vi "Mercury_GCS_All_VIs.vi"   [LabVIEW 2011]
doc: "This VI contains all high level and low level VIs valid for Mercury_GCS. See diagram for a survey of all Mercury_GCS high level and low level VIs. Menu / Browse / Show VI Hierarchy will show the file paths of the VIs. Global Variables are shown as Control as well as Indicator."
uses:
  Low Level/General command.llb/Controller names.ctl
  Low Level/Communication.llb/Available DLL interfaces.ctl
  Low Level/Communication.llb/Available DLLs.ctl
  Low Level/Communication.llb/Available interfaces.ctl
  Low Level/Communication.llb/Termination character.ctl
  Low Level/Analog control.llb/Available Analog Commands.ctl
  Low Level/Communication.llb/Global1.vi
  Low Level/General command.llb/Global2 (Array).vi
  Low Level/Communication.llb/Global DaisyChain.vi
  Low Level/Analog control.llb/Global Analog.vi
  Low Level/Support.llb/Unbunde/bundle interface clusters for PI Terminal.vi
panel:
  # "PI Mercury_GCS \nLabVIEW driver set"
  # "This VI contains all high level and low level VIs valid for Mercury_GCS. See diagram for a\nsurvey of all Mercury_GCS high level and low level VIs. Menu / Browse / Show VI \nhierarchy will show the file paths of the VIs. Global Variables are shown as Control as \nwell as Indicator."
types:
  T1 = typedef "Available Analog Commands.ctl" = enum16{"INITIALIZE", "VOL?", "VOL ", "CLOSE", "MOV", "POS?", "VCO", "VCO?", "WAIT_WF", "TMN?", "TMX?", "VEL", "VEL?", "SAI?", "MVR", "ERR?", "#24", "STP", "*IDN?", "#5", "STE", "DRR?", "W_Wave", "HLP?", "W/R_Wave"}
  T2 = typedef "Termination character.ctl" = enum16{"LF", "CR", "LFCR", "CRLF"}
  T3 = typedef "Available interfaces.ctl" = u16
  T4 = typedef "Available DLLs.ctl" = u16
  T5 = typedef "Available DLL interfaces.ctl" = u16
  T6 = typedef "Controller names.ctl" = enum16{"None", "Analog", "C-702", "C-843", "C-843.PM", "C-844", "C-848", "C-865", "C-866", "C-867", "C-880", "E-516", "E-517", "E-709", "E-710", "E-712", "E-725", "E-753", "E-755", "E-761", "E-816", "E-861", "F-206", "M-840", "M-850", "M-8X0", "Mercury", "Mercury_GCS"}
  T7 = cluster{"Conversion factor":dbl[], "Velocity":dbl[], "Velocity control mode":bool, "AO.Resolution":dbl, "Lower voltage limit (V)":dbl, "Upper voltage limit (V)":dbl, "AO_WF_T (s)":dbl, "AI Sample Rate":dbl, "AI Samples/Channel":i32, "Hyperbit":bool, "Offset (V)":dbl[], "Hyperbit StayOnPos":bool, "Gain (V)":dbl[], "Bit rate (Hz)":dbl, "PWM rate (Hz)":dbl, "HyperBit Password":string, "AO.MaxRate":dbl, "Conversion offset":dbl[]}[]
  T8 = cluster{"No. of devices":i32, "Port ID":i32, "Devices":string[], "Description":string}[]
  T9 = cluster{"Conn. axes":string[], "Controller name":T6}[]
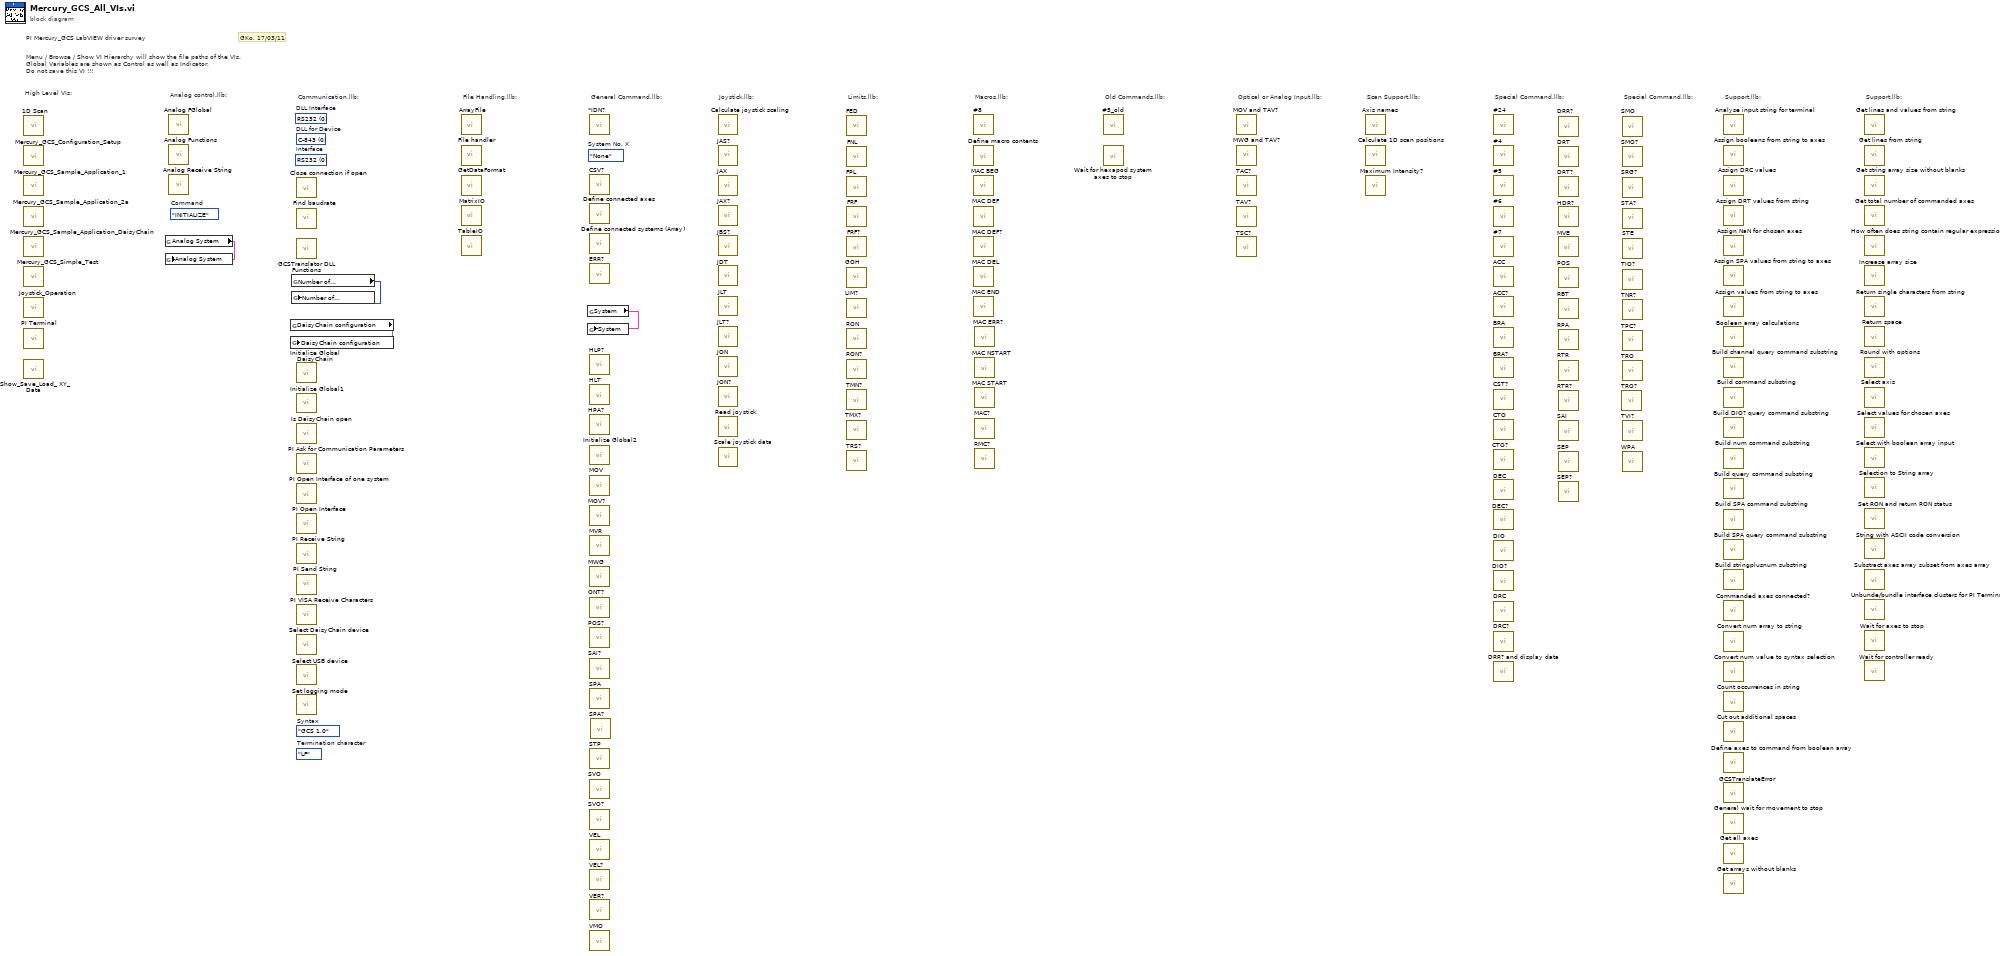
[diagram p0: block diagram]
diagram:
  (unwired) enum16{"GCS 1.0", "GCS 2.0"}."GCS 1.0"  # Syntax
  (unwired) Available_Analog_Commands."INITIALIZE"  # Command
  (unwired) Termination_character."LF"  # Termination character
  (unwired) T3 0 items=["RS232", "GPIB", "DLL", "TCP-IP"]  # Interface
  (unwired) T4 0 items=["C-843", "C-844", "E-710", "C-843.PM", "C-865", "E-761", "Mercury", "E-755", "E-753", "C-866", "E-712", "E-725", "E-861", "C-867", "E-517"]  # DLL for Device
  (unwired) T5 0 items=["RS232", "GPIB", "Board", "TCP-IP", "USB"]  # DLL Interface
  (unwired) Controller_names."None"  # System No. X
  # "GKo, 17/03/11"
  # "High Level VIs:"
  # "Analog control.llb:"
  # "Support.llb:"
  # "Special Command.llb:"
  # "Support.llb:"
  # "Special Command.llb:"
  # "Scan Support.llb:"
  # "Optical or Analog Input.llb:"
  # "Old Commands.llb:"
  # "Macros.llb:"
  # "Limits.llb:"
  # "Joystick.llb:"
  # "General Command.llb:"
  # "File Handling.llb:"
  # "Menu / Browse / Show VI Hierarchy will show the file paths of the VIs. \nGlobal Variables are shown as Control as well as Indicator.\nDo not save this VI !!!"
  # "PI Mercury_GCS LabVIEW driver survey"
  # "Communication.llb:"
  n1 = call "1D Scan.vi"() -> ()  [unwired: 23 in, 5 out]
  n2 = call "Mercury_GCS_Configuration_Setup.vi"() -> ()  [unwired: 13 in, 7 out]
  n3 = call "Mercury_GCS_Sample_Application_1.vi"() -> ()  [unwired: 1 in]
  n4 = call "Mercury_GCS_Sample_Application_2a.vi"() -> ()  [unwired: 15 in, 1 out]
  n5 = call "Mercury_GCS_Sample_Application_DaisyChain.vi"() -> ()  [unwired: 15 in, 1 out]
  n6 = call "Mercury_GCS_Simple_Test.vi"() -> ()  [unwired: 20 in]
  n7 = call "Joystick_Operation.vi"() -> ()  [unwired: 19 in, 1 out]
  n8 = call "PI Terminal.vi"() -> ()  [unwired: 20 in]
  n9 = call "Show_Save_Load_ XY_Data.vi"() -> ()  [unwired: 19 in, 1 out]
  n10 = global read "Global Analog.vi" "Analog System"() -> (w1:T7)
  n11 = global write "Global Analog.vi" "Analog System"(w1) -> ()
  n12 = call "Analog FGlobal.vi"() -> ()  [unwired: 19 in, 1 out]
  n13 = call "Analog Functions.vi"() -> ()  [unwired: 17 in, 3 out]
  n14 = call "Analog Receive String.vi"() -> ()  [unwired: 18 in, 2 out]
  n15 = global read "Global DaisyChain.vi" "DaisyChain configuration"() -> (w2:T8)
  n16 = global write "Global DaisyChain.vi" "DaisyChain configuration"(w2) -> ()
  n17 = global read "Global1.vi" "Number of\nsystems"() -> (w4:i32)
  n18 = global write "Global1.vi" "Number of\nsystems"(w4) -> ()
  n19 = call "Close connection if open.vi"() -> ()  [unwired: 18 in, 2 out]
  n20 = call "Find baudrate.vi"() -> ()  [unwired: 17 in, 3 out]
  n21 = call "GCSTranslator DLL Functions.vi"() -> ()  [unwired: 15 in, 5 out]
  n22 = call "Initialize Global DaisyChain.vi"() -> ()  [unwired: 19 in, 1 out]
  n23 = call "Initialize Global1.vi"() -> ()  [unwired: 19 in, 1 out]
  n24 = call "Is DaisyChain open.vi"() -> ()  [unwired: 17 in, 3 out]
  n25 = call "PI Ask for Communication Parameters.vi"() -> ()  [unwired: 12 in, 8 out]
  n26 = call "PI Open Interface of one system.vi"() -> ()  [unwired: 18 in, 2 out]
  n27 = call "PI Open Interface.vi"() -> ()  [unwired: 18 in, 2 out]
  n28 = call "PI Receive String.vi"() -> ()  [unwired: 17 in, 3 out]
  n29 = call "PI Send String.vi"() -> ()  [unwired: 19 in, 1 out]
  n30 = call "PI VISA Receive Characters.vi"() -> ()  [unwired: 17 in, 3 out]
  n31 = call "Select DaisyChain device.vi"() -> ()  [unwired: 17 in, 3 out]
  n32 = call "Select USB device.vi"() -> ()  [unwired: 17 in, 3 out]
  n33 = call "Set logging mode.vi"() -> ()  [unwired: 19 in, 1 out]
  n34 = call "ArrayFile.vi"() -> ()  [unwired: 18 in, 2 out]
  n35 = call "File handler.vi"() -> ()  [unwired: 17 in, 3 out]
  n36 = call "GetDataFormat.vi"() -> ()  [unwired: 12 in, 8 out]
  n37 = call "MatrixIO.vi"() -> ()  [unwired: 13 in, 7 out]
  n38 = call "TableIO.vi"() -> ()  [unwired: 14 in, 6 out]
  n39 = global read "Global2 (Array).vi" "System"() -> (w3:T9)
  n40 = global write "Global2 (Array).vi" "System"(w3) -> ()
  n41 = call "*IDN?.vi"() -> ()  [unwired: 18 in, 2 out]
  n42 = call "CSV?.vi"() -> ()  [unwired: 18 in, 2 out]
  n43 = call "Define connected axes.vi"() -> ()  [unwired: 18 in, 2 out]
  n44 = call "Define connected systems (Array).vi"() -> ()  [unwired: 19 in, 1 out]
  n45 = call "ERR?.vi"() -> ()  [unwired: 18 in, 2 out]
  n46 = call "HLP?.vi"() -> ()  [unwired: 18 in, 2 out]
  n47 = call "HLT.vi"() -> ()  [unwired: 19 in, 1 out]
  n48 = call "HPA?.vi"() -> ()  [unwired: 18 in, 2 out]
  n49 = call "Initialize Global2.vi"() -> ()  [unwired: 19 in, 1 out]
  n50 = call "MOV.vi"() -> ()  [unwired: 19 in, 1 out]
  n51 = call "MOV?.vi"() -> ()  [unwired: 18 in, 2 out]
  n52 = call "MVR.vi"() -> ()  [unwired: 19 in, 1 out]
  n53 = call "MWG.vi"() -> ()  [unwired: 19 in, 1 out]
  n54 = call "ONT?.vi"() -> ()  [unwired: 18 in, 2 out]
  n55 = call "POS?.vi"() -> ()  [unwired: 18 in, 2 out]
  n56 = call "SAI?.vi"() -> ()  [unwired: 18 in, 2 out]
  n57 = call "SPA.vi"() -> ()  [unwired: 18 in, 2 out]
  n58 = call "STP.vi"() -> ()  [unwired: 19 in, 1 out]
  n59 = call "SVO.vi"() -> ()  [unwired: 19 in, 1 out]
  n60 = call "SVO?.vi"() -> ()  [unwired: 18 in, 2 out]
  n61 = call "VEL.vi"() -> ()  [unwired: 18 in, 2 out]
  n62 = call "VEL?.vi"() -> ()  [unwired: 18 in, 2 out]
  n63 = call "VER?.vi"() -> ()  [unwired: 18 in, 2 out]
  n64 = call "VMO.vi"() -> ()  [unwired: 18 in, 2 out]
  n65 = call "SPA?.vi"() -> ()  [unwired: 14 in, 6 out]
  n66 = call "Calculate joystick scaling.vi"() -> ()  [unwired: 10 in, 10 out]
  n67 = call "JAS?.vi"() -> ()  [unwired: 18 in, 2 out]
  n68 = call "JAX.vi"() -> ()  [unwired: 19 in, 1 out]
  n69 = call "JAX?.vi"() -> ()  [unwired: 18 in, 2 out]
  n70 = call "JBS?.vi"() -> ()  [unwired: 18 in, 2 out]
  n71 = call "JDT.vi"() -> ()  [unwired: 18 in, 2 out]
  n72 = call "JLT.vi"() -> ()  [unwired: 18 in, 2 out]
  n73 = call "JLT?.vi"() -> ()  [unwired: 17 in, 3 out]
  n74 = call "JON.vi"() -> ()  [unwired: 18 in, 2 out]
  n75 = call "JON?.vi"() -> ()  [unwired: 18 in, 2 out]
  n76 = call "Read joystick.vi"() -> ()  [unwired: 15 in, 5 out]
  n77 = call "Scale joystick data.vi"() -> ()  [unwired: 18 in, 2 out]
  n78 = call "FED.vi"() -> ()  [unwired: 19 in, 1 out]
  n79 = call "FNL.vi"() -> ()  [unwired: 19 in, 1 out]
  n80 = call "FPL.vi"() -> ()  [unwired: 19 in, 1 out]
  n81 = call "FRF.vi"() -> ()  [unwired: 19 in, 1 out]
  n82 = call "FRF?.vi"() -> ()  [unwired: 18 in, 2 out]
  n83 = call "GOH.vi"() -> ()  [unwired: 19 in, 1 out]
  n84 = call "LIM?.vi"() -> ()  [unwired: 18 in, 2 out]
  n85 = call "RON.vi"() -> ()  [unwired: 19 in, 1 out]
  n86 = call "RON?.vi"() -> ()  [unwired: 18 in, 2 out]
  n87 = call "TMN?.vi"() -> ()  [unwired: 18 in, 2 out]
  n88 = call "TMX?.vi"() -> ()  [unwired: 18 in, 2 out]
  n89 = call "TRS?.vi"() -> ()  [unwired: 18 in, 2 out]
  n90 = call "#8.vi"() -> ()  [unwired: 17 in, 3 out]
  n91 = call "Define macro contents.vi"() -> ()  [unwired: 19 in, 1 out]
  n92 = call "MAC BEG.vi"() -> ()  [unwired: 19 in, 1 out]
  n93 = call "MAC DEF.vi"() -> ()  [unwired: 19 in, 1 out]
  n94 = call "MAC DEF?.vi"() -> ()  [unwired: 18 in, 2 out]
  n95 = call "MAC DEL.vi"() -> ()  [unwired: 18 in, 2 out]
  n96 = call "MAC END.vi"() -> ()  [unwired: 19 in, 1 out]
  n97 = call "MAC ERR?.vi"() -> ()  [unwired: 18 in, 2 out]
  n98 = call "MAC NSTART.vi"() -> ()  [unwired: 19 in, 1 out]
  n99 = call "MAC START.vi"() -> ()  [unwired: 19 in, 1 out]
  n100 = call "MAC?.vi"() -> ()  [unwired: 18 in, 2 out]
  n101 = call "RMC?.vi"() -> ()  [unwired: 18 in, 2 out]
  n102 = call "#5_old.vi"() -> ()  [unwired: 16 in, 4 out]
  n103 = call "Wait for hexapod system axes to stop.vi"() -> ()  [unwired: 18 in, 2 out]
  n104 = call "MOV and TAV?.vi"() -> ()  [unwired: 18 in, 2 out]
  n105 = call "MWG and TAV?.vi"() -> ()  [unwired: 18 in, 2 out]
  n106 = call "TAC?.vi"() -> ()  [unwired: 18 in, 2 out]
  n107 = call "TAV?.vi"() -> ()  [unwired: 16 in, 4 out]
  n108 = call "TSC?.vi"() -> ()  [unwired: 18 in, 2 out]
  n109 = call "Axis names.vi"() -> ()  [unwired: 17 in, 3 out]
  n110 = call "Calculate 1D scan positions.vi"() -> ()  [unwired: 15 in, 5 out]
  n111 = call "Maximum Intensity?.vi"() -> ()  [unwired: 16 in, 4 out]
  n112 = call "CTO.vi"() -> ()  [unwired: 18 in, 2 out]
  n113 = call "CTO?.vi"() -> ()  [unwired: 16 in, 4 out]
  n114 = call "#24.vi"() -> ()  [unwired: 19 in, 1 out]
  n115 = call "#4.vi"() -> ()  [unwired: 18 in, 2 out]
  n116 = call "#5.vi"() -> ()  [unwired: 18 in, 2 out]
  n117 = call "#6.vi"() -> ()  [unwired: 18 in, 2 out]
  n118 = call "#7.vi"() -> ()  [unwired: 17 in, 3 out]
  n119 = call "ACC.vi"() -> ()  [unwired: 18 in, 2 out]
  n120 = call "ACC?.vi"() -> ()  [unwired: 18 in, 2 out]
  n121 = call "BRA.vi"() -> ()  [unwired: 19 in, 1 out]
  n122 = call "BRA?.vi"() -> ()  [unwired: 17 in, 3 out]
  n123 = call "CST?.vi"() -> ()  [unwired: 18 in, 2 out]
  n124 = call "DEC.vi"() -> ()  [unwired: 18 in, 2 out]
  n125 = call "DEC?.vi"() -> ()  [unwired: 18 in, 2 out]
  n126 = call "DIO.vi"() -> ()  [unwired: 19 in, 1 out]
  n127 = call "DIO?.vi"() -> ()  [unwired: 18 in, 2 out]
  n128 = call "DRC.vi"() -> ()  [unwired: 18 in, 2 out]
  n129 = call "DRC?.vi"() -> ()  [unwired: 16 in, 4 out]
  n130 = call "DRR? and display data.vi"() -> ()  [unwired: 16 in, 4 out]
  n131 = call "DRR?.vi"() -> ()  [unwired: 16 in, 4 out]
  n132 = call "DRT.vi"() -> ()  [unwired: 18 in, 2 out]
  n133 = call "DRT?.vi"() -> ()  [unwired: 17 in, 3 out]
  n134 = call "HDR?.vi"() -> ()  [unwired: 16 in, 4 out]
  n135 = call "MVE.vi"() -> ()  [unwired: 19 in, 1 out]
  n136 = call "POS.vi"() -> ()  [unwired: 19 in, 1 out]
  n137 = call "RBT.vi"() -> ()  [unwired: 19 in, 1 out]
  n138 = call "RPA.vi"() -> ()  [unwired: 18 in, 2 out]
  n139 = call "RTR.vi"() -> ()  [unwired: 18 in, 2 out]
  n140 = call "RTR?.vi"() -> ()  [unwired: 18 in, 2 out]
  n141 = call "SAI.vi"() -> ()  [unwired: 19 in, 1 out]
  n142 = call "SEP.vi"() -> ()  [unwired: 18 in, 2 out]
  n143 = call "SEP?.vi"() -> ()  [unwired: 14 in, 6 out]
  n144 = call "TRO?.vi"() -> ()  [unwired: 18 in, 2 out]
  n145 = call "SMO.vi"() -> ()  [unwired: 18 in, 2 out]
  n146 = call "SMO?.vi"() -> ()  [unwired: 18 in, 2 out]
  n147 = call "SRG?.vi"() -> ()  [unwired: 18 in, 2 out]
  n148 = call "STA?.vi"() -> ()  [unwired: 18 in, 2 out]
  n149 = call "STE.vi"() -> ()  [unwired: 19 in, 1 out]
  n150 = call "TIO?.vi"() -> ()  [unwired: 17 in, 3 out]
  n151 = call "TNR?.vi"() -> ()  [unwired: 18 in, 2 out]
  n152 = call "TPC?.vi"() -> ()  [unwired: 18 in, 2 out]
  n153 = call "TRO.vi"() -> ()  [unwired: 19 in, 1 out]
  n154 = call "TVI?.vi"() -> ()  [unwired: 18 in, 2 out]
  n155 = call "WPA.vi"() -> ()  [unwired: 18 in, 2 out]
  n156 = call "Analyse input string for terminal.vi"() -> ()  [unwired: 17 in, 3 out]
  n157 = call "Assign booleans from string to axes.vi"() -> ()  [unwired: 18 in, 2 out]
  n158 = call "Assign DRC values.vi"() -> ()  [unwired: 14 in, 6 out]
  n159 = call "Assign DRT values from string.vi"() -> ()  [unwired: 14 in, 6 out]
  n160 = call "Assign NaN for chosen axes.vi"() -> ()  [unwired: 19 in, 1 out]
  n161 = call "Assign SPA values from string to axes.vi"() -> ()  [unwired: 14 in, 6 out]
  n162 = call "Assign values from string to axes.vi"() -> ()  [unwired: 16 in, 4 out]
  n163 = call "Boolean array calculations.vi"() -> ()  [unwired: 19 in, 1 out]
  n164 = call "Build channel query command substring.vi"() -> ()  [unwired: 16 in, 4 out]
  n165 = call "Build command substring.vi"() -> ()  [unwired: 19 in, 1 out]
  n166 = call "Build DIO? query command substring.vi"() -> ()  [unwired: 16 in, 4 out]
  n167 = call "Build num command substring.vi"() -> ()  [unwired: 19 in, 1 out]
  n168 = call "Build query command substring.vi"() -> ()  [unwired: 17 in, 3 out]
  n169 = call "Build SPA command substring.vi"() -> ()  [unwired: 19 in, 1 out]
  n170 = call "Build SPA query command substring.vi"() -> ()  [unwired: 18 in, 2 out]
  n171 = call "Build stringplusnum substring.vi"() -> ()  [unwired: 18 in, 2 out]
  n172 = call "Commanded axes connected?.vi"() -> ()  [unwired: 18 in, 2 out]
  n173 = call "Convert num array to string.vi"() -> ()  [unwired: 19 in, 1 out]
  n174 = call "Convert num value to syntax selection.vi"() -> ()  [unwired: 19 in, 1 out]
  n175 = call "Count occurrences in string.vi"() -> ()  [unwired: 19 in, 1 out]
  n176 = call "Cut out additional spaces.vi"() -> ()  [unwired: 19 in, 1 out]
  n177 = call "Define axes to command from boolean array.vi"() -> ()  [unwired: 17 in, 3 out]
  n178 = call "GCSTranslateError.vi"() -> ()  [unwired: 17 in, 3 out]
  n179 = call "General wait for movement to stop.vi"() -> ()  [unwired: 18 in, 2 out]
  n180 = call "Get all axes.vi"() -> ()  [unwired: 19 in, 1 out]
  n181 = call "Get arrays without blanks.vi"() -> ()  [unwired: 16 in, 4 out]
  n182 = call "Get lines and values from string.vi"() -> ()  [unwired: 17 in, 3 out]
  n183 = call "Get lines from string.vi"() -> ()  [unwired: 18 in, 2 out]
  n184 = call "Get string array size without blanks.vi"() -> ()  [unwired: 19 in, 1 out]
  n185 = call "Get total number of commanded axes.vi"() -> ()  [unwired: 16 in, 4 out]
  n186 = call "How often does string contain regular expression?.vi"() -> ()  [unwired: 19 in, 1 out]
  n187 = call "Increase array size.vi"() -> ()  [unwired: 19 in, 1 out]
  n188 = call "Return single characters from string.vi"() -> ()  [unwired: 18 in, 2 out]
  n189 = call "Return space.vi"() -> ()  [unwired: 18 in, 2 out]
  n190 = call "Round with options.vi"() -> ()  [unwired: 18 in, 2 out]
  n191 = call "Select axis.vi"() -> ()  [unwired: 17 in, 3 out]
  n192 = call "Select values for chosen axes.vi"() -> ()  [unwired: 17 in, 3 out]
  n193 = call "Select with boolean array input.vi"() -> ()  [unwired: 19 in, 1 out]
  n194 = call "Selection to String array.vi"() -> ()  [unwired: 19 in, 1 out]
  n195 = call "Set RON and return RON status.vi"() -> ()  [unwired: 17 in, 3 out]
  n196 = call "String with ASCII code conversion.vi"() -> ()  [unwired: 19 in, 1 out]
  n197 = call "Substract axes array subset from axes array.vi"() -> ()  [unwired: 18 in, 2 out]
  n198 = call "Unbunde/bundle interface clusters for PI Terminal.vi"() -> ()  [unwired: 13 in, 7 out]
  n199 = call "Wait for axes to stop.vi"() -> ()  [unwired: 18 in, 2 out]
  n200 = call "Wait for controller ready.vi"() -> ()  [unwired: 18 in, 2 out]
